vi "PyBD Tiles.vi"() -> ()   [LabVIEW 2016]
uses:
  VIs/uPythonX/uPythonX.xctl
panel:
  in  "Tiles":T1(xcontrol)={"VISA Refnum in"="ASRL96::INSTR", "Python Code"="'''\nhttps://pybd.io/hw/tile_sensa.html\n\ntwo different i2c addresses, 64 and 69 for temp and light\nLEDs on X2,3,4\n'''\n\nclass HDC2080:\n     def __init__(self, i2c, addr=64):\n          self.i2c = i2c\n          self.addr = addr\n\n     def is_ready(self):\n          return self.i2c.readfrom_mem(self.addr, 0x0f, 1)[0] & 1 == 0\n\n     def measure(self):\n          self.i2c.writeto_mem(self.addr, 0x0f, b'\\x01')\n\n     def temperature(self):\n          data = self.i2c.readfrom_mem(self.addr, 0x00, 2)\n          data = data[0] | data[1] << 8\n          return data / 0x10000 * 165 - 40\n\n     def humidity(self):\n          data = self.i2c.readfrom_mem(self.addr, 0x02, 2)\n          data = data[0] | data[1] << 8\n          return data / 0x10000 * 100\n          \nclass OPT3001:\n     def __init__(self, i2c, addr=69):\n          self.i2c = i2c\n          self.addr = addr\n\n     def is_ready(self):\n          return bool(self.i2c.readfrom_mem(self.addr, 0x01, 2)[1] & 0x80)\n\n     def measure(self):\n          self.i2c.writeto_mem(self.addr, 0x01, b'\\xca\\x10')\n\n     def lux(self):\n          data = self.i2c.readfrom_mem(self.addr, 0, 2)\n          return 0.01 * 2 ** (data[0] >> 4) * ((data[0] & 0x0f) << 8 | data[1])\n\n\nfrom machine import Pin, Signal\nimport utime\nimport machine, SystemLink\n\ni2c = machine.I2C('X')\nhdc = HDC2080(i2c)\nopt = OPT3001(i2c)\nled_b = Signal('X4', Pin.OUT, value=0, invert=True)\n\nfred2 = SystemLink.SystemLink('fred2','STRING')\nfred2.connect()\n\nwhile True:\n     hdc.measure()\n     opt.measure()\n     led_b.on()\n     while not hdc.is_ready():\n          machine.idle()\n     print(hdc.temperature(), hdc.humidity())\n     while not opt.is_ready():\n          machine.idle()\n     print(opt.lux())\n     if fred2.status():\n          fred2.put(str(hdc.temperature()))\n     led_b.off()\n     utime.sleep(1)"}
  in  "SystemLink":T1(xcontrol)={"VISA Refnum in"="ASRL96::INSTR", "Python Code"="'''\nThis talks to SystemLink \n\nfred2 = SystemLink('fred2','STRING')\nfred2.connect()\nfred2.status()\nfred2.get()\na,b = fred2.put('test')\nif b == 'Tag Value Updated':\n     print('success')\n     \n'''\nimport machine, network, ubinascii, ujson, urequests, utime\n     \nclass SystemLink(object):\n     def __init__(self,tag,type = 'STRING'):\n          self.WiFi = network.WLAN()\n          mac = ubinascii.hexlify(network.WLAN().config(\"mac\"),\":\").decode()\n          print(\"MAC address: \" + mac)\n          self.SSID = 'Rogers'\n          self.passwd = 's0meth1ng'\n          self.Key = \"dYy-vDU9TXxDCy2QG3jO4J0s1-QUyYs6sO1xPd1oKQ\"\n          self.tag = tag\n          self.type = type\n          self.url_tag = \"https://api.systemlinkcloud.com/nitag/v2/tags/\" + tag\n          self.url_value = self.url_tag + '/values/current'\n          self.headers = {\"Accept\":\"application/json\",\"x-ni-api-key\":self.Key}\n\n     def connect(self):\n          status = True\n          if not self.WiFi.isconnected():\n               print (\"Connecting ..\")\n               self.WiFi.active(True)\n               self.WiFi.connect(self.SSID,self.passwd)\n               i=0\n               while i < 25 and not self.WiFi.isconnected():\n                    utime.sleep_ms(200)\n                    i=i+1\n               if self.WiFi.isconnected():\n                    print (\"Connection succeeded\")\n               else:\n                    print (\"Connection failed\")\n                    status = False\n          return status\n                    \n     def status(self):\n          return self.WiFi.isconnected()\n                    \n     def put(self,value):\n          propName={\"type\":self.type,\"path\":self.tag}\n          propValue = {\"value\":{\"type\":self.type,\"value\":value}}\n\n          try:\n               setTag = urequests.put(self.url_tag,headers=self.headers,json=propName).text\n               setValue = urequests.put(self.url_value,headers=self.headers,json=propValue).text\n          except:\n               setTag = 'error'\n               setValue = 'error'\n          return setTag,setValue\n\n     def get(self):\n          try:\n               value = urequests.get(self.url_value,headers=self.headers).text\n               data = ujson.loads(value)\n               result = data.get(\"value\").get(\"value\")\n               print (\"value = \",result)\n          except:\n               result = 'error'\n          return result\n          "}
  in  "TILE-SENSA":T1(xcontrol)={"VISA Refnum in"="ASRL96::INSTR", "Python Code"="'''\nhttps://pybd.io/hw/tile_sensa.html\n\ntwo different i2c addresses, 64 and 69 for temp and light\nLEDs on X2,3,4\n'''\n\n\nfrom machine import Pin, Signal\nimport utime\n\nled_r = Signal('X2', Pin.OUT, value=0, invert=True)\nled_g = Signal('X3', Pin.OUT, value=0, invert=True)\nled_b = Signal('X4', Pin.OUT, value=0, invert=True)\n\nled_r.on()\nutime.sleep(1)\nled_r.off()\nled_g.on()\nutime.sleep(1)\nled_g.off()\nled_b.on()\nutime.sleep(1)\nled_b.off()\n\nclass HDC2080:\n     def __init__(self, i2c, addr=64):\n          self.i2c = i2c\n          self.addr = addr\n\n     def is_ready(self):\n          return self.i2c.readfrom_mem(self.addr, 0x0f, 1)[0] & 1 == 0\n\n     def measure(self):\n          self.i2c.writeto_mem(self.addr, 0x0f, b'\\x01')\n\n     def temperature(self):\n          data = self.i2c.readfrom_mem(self.addr, 0x00, 2)\n          data = data[0] | data[1] << 8\n          return data / 0x10000 * 165 - 40\n\n     def humidity(self):\n          data = self.i2c.readfrom_mem(self.addr, 0x02, 2)\n          data = data[0] | data[1] << 8\n          return data / 0x10000 * 100\n          \nclass OPT3001:\n     def __init__(self, i2c, addr=69):\n          self.i2c = i2c\n          self.addr = addr\n\n     def is_ready(self):\n          return bool(self.i2c.readfrom_mem(self.addr, 0x01, 2)[1] & 0x80)\n\n     def measure(self):\n          self.i2c.writeto_mem(self.addr, 0x01, b'\\xca\\x10')\n\n     def lux(self):\n          data = self.i2c.readfrom_mem(self.addr, 0, 2)\n          return 0.01 * 2 ** (data[0] >> 4) * ((data[0] & 0x0f) << 8 | data[1])\n\nimport machine\ni2c = machine.I2C('X')\nhdc = HDC2080(i2c)\nopt = OPT3001(i2c)\nwhile True:\n     hdc.measure()\n     opt.measure()\n     while not hdc.is_ready():\n          machine.idle()\n     print(hdc.temperature(), hdc.humidity())\n     while not opt.is_ready():\n          machine.idle()\n     print(opt.lux())"}
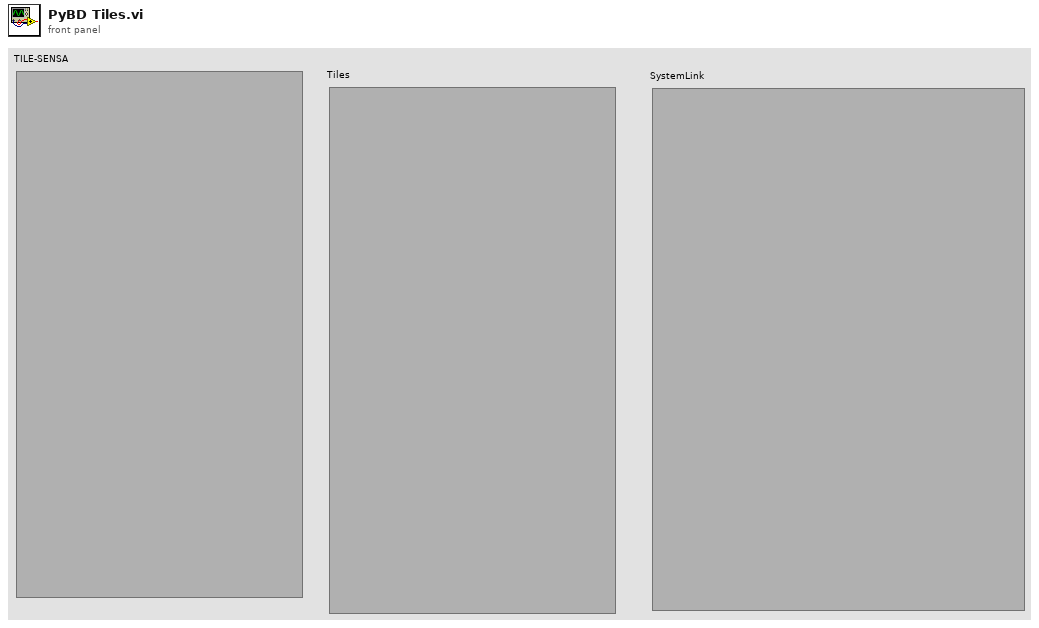
[diagram p1: front panel]
types:
  T1 = cluster{"VISA Refnum in":refnum<visa-resource-name>, "Python Code":string}
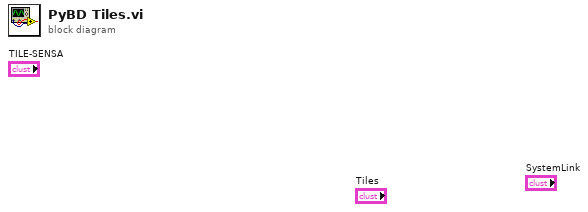
[diagram p0: block diagram]
diagram:
